vi "Send Remote Message.vi"(5 "Target Task (None)":string, 7 "Target Name":string, 8 "error in (no error)":errorcluster, 9 "Message Type":string, 10 "Message":refnum<class "Message.lvclass">, 11 "VolatusAPI in":refnum<class "VolatusAPI.lvclass">) -> (0 "error out":errorcluster, 3 "VolatusAPI out":refnum<class "VolatusAPI.lvclass">)   [LabVIEW 2020, in "Volatus.lvlib" / "VolatusAPI.lvclass"]
uses:
  VolatusAPI.lvclass
  VolatusAPI.lvclass/VolatusAPI.ctl
  lv-vecto/Vecto/TCPMessageService/TCPMessageAPI.lvclass
  lv-protoc/LV-Proto/Message/Message.lvclass
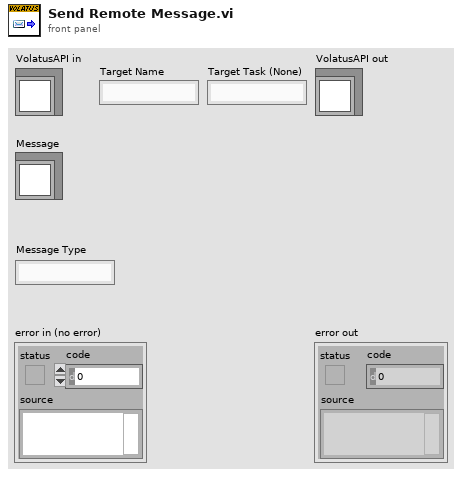
[diagram p1: front panel]
types:
  T1 = typedef "VolatusConfig.lvlib/Target Info.ctl" = cluster{"ID":u32, "Type":T2}
  T2 = typedef "VolatusConfig.lvlib/Target Type.ctl" = enum16{"Unknown", "Node", "Group"}
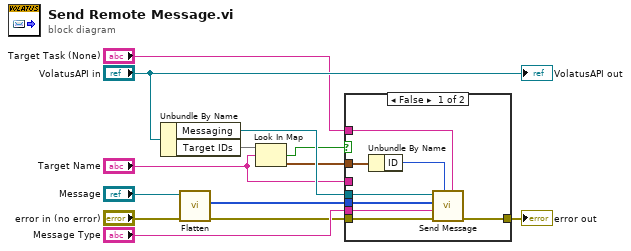
[diagram p0: block diagram]
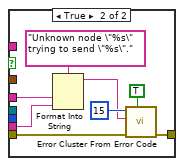
[diagram p2: hidden frame]
diagram:
  n1 = Unbundle By Name("VolatusAPI in") -> ("Messaging"=w12:refnum<class "TCPMessageAPI.lvclass">, "Target IDs"=w4:map{string, T1})
  n2 = call-dynamic "Flatten.vi"("error in (no error)"="error in (no error)", "Message in"="Message") -> ("error out"=w6:errorcluster, "Buffer"=w5:u8[])  [unwired: 7 in, 1 out]
  n3 = Look In Map(map=w4, key="Target Name") -> (key not found?=w3:bool, value=w2:T1)  [unwired: 1 in]
  n4 = case shown="False" w3 {
    tunnel: w12 -> [w21 _]
    tunnel: "Message Type" -> [w20 w22]
    tunnel: "Target Task (None)" -> [w19 _]
    tunnel: [w18 w28] -> w9
    tunnel: w6 -> [w17 w29]
    tunnel: w5 -> [w16 _]
    tunnel: w2 -> [w15 _]
    tunnel: "Target Name" -> [_ w26]
    frame False {
      n5 = Unbundle By Name(w15) -> ("ID"=w14:u32)
      n6 = call "Send Message.vi"("Target Task"=w19, "Target ID"=w14, "error in (no error)"=w17, "Type"=w20, "Payload"=w16, "TCPMessageService in"=w21) -> ("error out"=w18:errorcluster)  [unwired: 4 in, 1 out]
    }
    frame True {
      n7 = Format Into String(format string="Unknown node \"%s\" trying to send \"%s\".", w26, w22) -> (resulting string=w23:string)  [unwired: 2 in, 1 out]
      n8 = call <vilib>:"Error Cluster From Error Code.vi"("show call chain? (False)"=TRUE, "error in (no error)"=w29, "error message (\"\")"=w23, "error code (0)"=15) -> ("error out"=w28:errorcluster)  [unwired: 5 in]
    }
  }
  "error out" <- w9
  "VolatusAPI out" <- "VolatusAPI in"
